vi "Write.vi"(0 "element":string) -> (1 "previous element":string, 2 "channel":T1)   [LabVIEW 2020, in "Tag-str.lvlib"]
doc: "Writes a value to a Tag channel."
uses:
  <extravilib>/ChannelInstances/Tag-str.lvlib
  <extravilib>/ChannelInstances/Tag-str/))Channel.ctl
  <extravilib>/ChannelInstances/Tag-str/Endpoint.vi
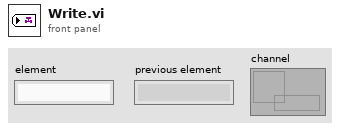
[diagram p1: front panel]
types:
  T1 = typedef "Tag-str.lvlib/))Channel.ctl" = refnum<queue>
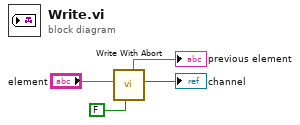
[diagram p0: block diagram]
diagram:
  n1 = call <extravilib>:"Write With Abort.vi"("abort"=FALSE, "element"="element") -> ("channel"=→"channel":T1, "previous element"=→"previous element":string)  [unwired: 7 in, 1 out]
